vi "Assert in Report.vi"(7 "VI:s to Measure":cluster{"element":path, "value":dbl}[](array[cluster])=[{"element"=path "My VI.vi", "value"=1.0}], 10 "Regular Expression":string, 11 "Coverage Report Test in":refnum<class "Coverage Report Test.lvclass">) -> (0 "error out":errorcluster, 3 "Coverage Report Test out":refnum<class "Coverage Report Test.lvclass">)   [LabVIEW 2020, in "Coverage Report Test.lvclass"]
uses:
  Coverage Report Test.lvclass
  C:/Program Files (x86)/National Instruments/LabVIEW 2020/vi.lib/Astemes/LUnit/Test Case.lvclass
  Coverage Report Test.lvclass/Coverage Report Test.ctl
  <vilib>/Astemes/LUnit/Test Case.lvclass/Test Case.ctl
  <vilib>/Astemes/LUnit/Palette/Pass If.vi
  <vilib>/Astemes/LUnit/Core/LUnit Test Case/Private/Append Fail Result.vi
  <vilib>/Astemes/LUnit/Core/LUnit Test Case/Private/Append Pass Result.vi
  <vilib>/Astemes/LUnit/Core/LUnit Test Case/Private/Run In UI.vi
  <vilib>/Utility/error.llb/Clear Errors.vi
  source/Coverage Report/Coverage Report.lvclass
  <vilib>/Astemes/LUnit/Palette/Advanced Assertions/LUnit Advanced Assertions.lvlib
panel:
  out "text":string
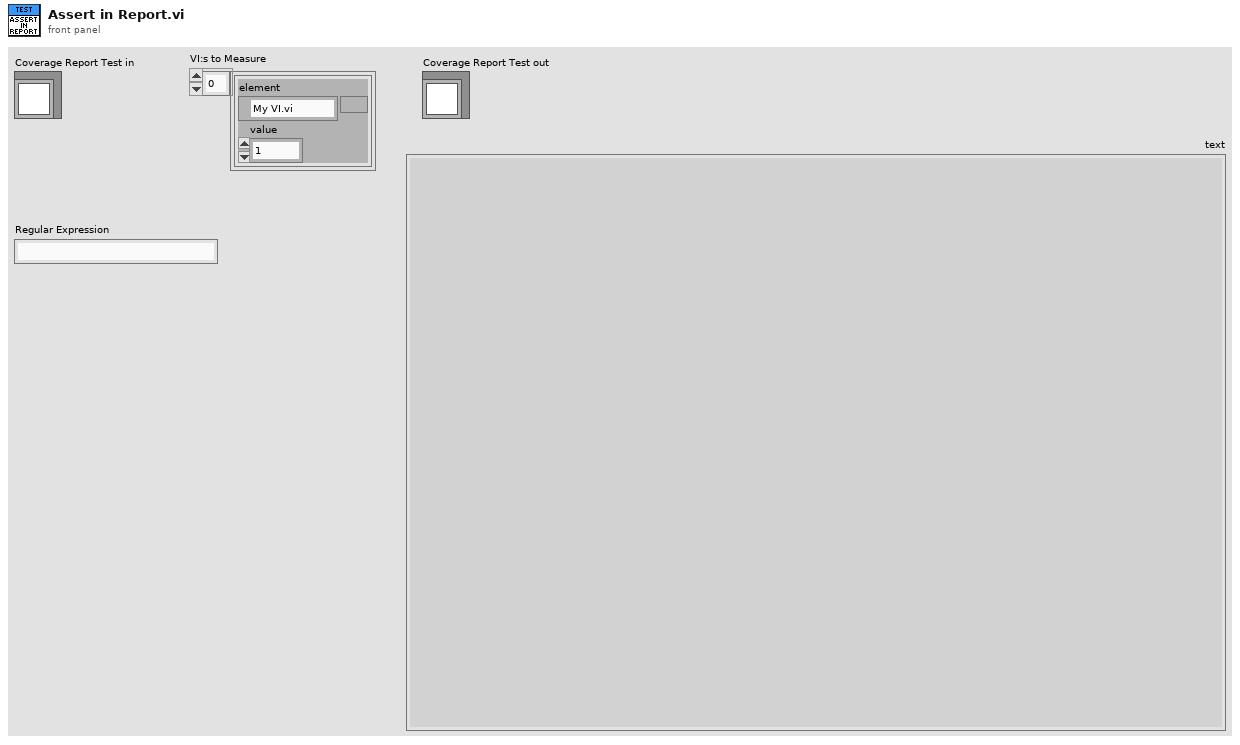
[diagram p1: front panel]
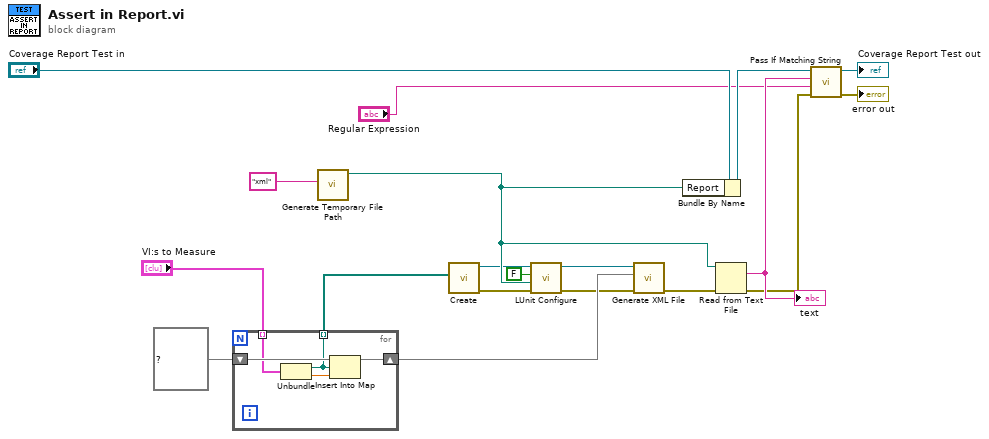
[diagram p0: block diagram]
diagram:
  n1 = for {
    shift-right: [w23] -> w17
    shift-left: map{path, dbl} {} ("Code Coverage") -> [w24]
    tunnel: "VI:s to Measure" -> [w22] mode=indexing
    tunnel: [w20] -> w1 mode=indexing
    n2 = Unbundle(w22) -> ("element"=w20:path, "value"=w21:dbl)
    n3 = Insert Into Map(map in=w24, key=w20, value=w21) -> (map out=w23:map{path, dbl})  [unwired: 2 out]
  }
  n4 = call <vilib>:"Generate Temporary File Path.vi"("Temporary File Extension (tmp)"="xml") -> ("Unique Temporary File Path"=w19:path)  [unwired: 9 in, 1 out]
  n5 = call "Create.vi"("VI:s to Measure"=w1) -> ("error out"=w8:errorcluster, "Coverage Report"=w7:refnum<class "Coverage Report.lvclass">)  [unwired: 9 in]
  n6 = call-dynamic "LUnit Configure.vi"("error in (no error)"=w8, "Default Path"=w19, "Interactive?"=FALSE, "Coverage Report In"=w7) -> ("error out"=w11:errorcluster, "Coverage Report Out"=w10:refnum<class "Coverage Report.lvclass">)  [unwired: 6 in]
  n7 = call "Generate XML File.vi"("error in (no error)"=w11, "Code Coverage"=w17, "Coverage Report in"=w10) -> ("error out"=w12:errorcluster)  [unwired: 6 in, 2 out]
  n8 = Bundle By Name(cluster="Coverage Report Test in", "Report"=w19) -> (w18:refnum<class "Coverage Report Test.lvclass">)
  n9 = Read from Text File(file (use dialog)=w19, error in=w12) -> (text=w14:string, error out=w13:errorcluster)  [unwired: 2 in, 2 out]
  "text" <- w14
  n10 = call <vilib>:"Pass If Matching String.vi"("error in (no error)"=w13, "Regular Expression"="Regular Expression", "String"=w14, "LUnit Test Case In"=w18) -> ("error out"=→"error out":errorcluster, "LUnit Test Case Out"=→"Coverage Report Test out":refnum<class "Coverage Report Test.lvclass">)  [unwired: 6 in]
